vi "Get position.vi"(0 "Zaber":T1={"Serial port handle"="", "Axis"="", "Controller #"=0, "Min position"=0.0, "Max position"=0.0, "Min velocity"=0.0, "Max velocity"=0.0, "Firmware"="", "Device ID"=0, "Variable event"=refnum, "Variable ref"=refnum, "Resolution, usteps/step"=0, "Serial port semaphore"=refnum, "Joystick buttons"={"MinDir"=1, "MaxDir"=2, "MedSpeed"=5, "HighSpeed"=6}} {"Joystick buttons"."HighSpeed" min=1 max=25 step=1; "Joystick buttons"."MedSpeed" min=1 max=25 step=1; "Joystick buttons"."MaxDir" min=1 max=25 step=1; "Joystick buttons"."MinDir" min=1 max=25 step=1}, 5 "error in":errorcluster) -> (11 "Command time, ms":u32, 14 "Zaber out":T1={"Serial port handle"="", "Axis"="", "Controller #"=0, "Min position"=0.0, "Max position"=0.0, "Min velocity"=0.0, "Max velocity"=0.0, "Firmware"="", "Device ID"=0, "Variable event"=refnum, "Variable ref"=refnum, "Resolution, usteps/step"=0, "Serial port semaphore"=refnum, "Joystick buttons"={"MinDir"=1, "MaxDir"=2, "MedSpeed"=5, "HighSpeed"=6}} {"Joystick buttons"."HighSpeed" min=1 max=25 step=1; "Joystick buttons"."MedSpeed" min=1 max=25 step=1; "Joystick buttons"."MaxDir" min=1 max=25 step=1; "Joystick buttons"."MinDir" min=1 max=25 step=1}, 15 "Position, usteps":i32, 16 "PositionRb":dbl caption="Position, mm", 19 "error out":errorcluster)   [LabVIEW 2018]
uses:
  Zaber.ctl
  GenericDataEvent/GenericEvent.ctl
  ZaberVariables.ctl
  CommandZaber.ctl
  GenericDataEvent/GenericData.ctl
panel:
  out "x-y 2":u32
  out "x-y":u32
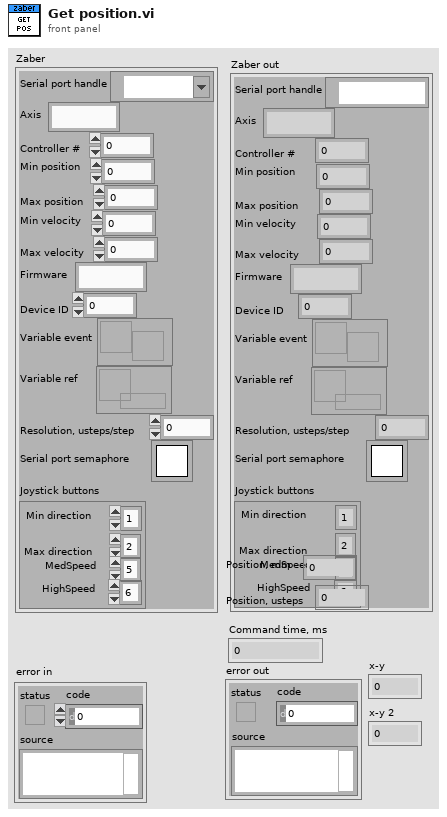
[diagram p1: front panel]
types:
  T1 = typedef "Zaber.ctl" = cluster{"Serial port handle":refnum<visa-resource-name>, "Axis":string, "Controller #":u8, "Min position":dbl, "Max position":dbl, "Min velocity":dbl, "Max velocity":dbl, "Firmware":string, "Device ID":i32, "Variable event":T2, "Variable ref":refnum<data-value>, "Resolution, usteps/step":i32, "Serial port semaphore":T3, "Joystick buttons":cluster{"MinDir":i32, "MaxDir":i32, "MedSpeed":i32, "HighSpeed":i32}}
  T2 = typedef "GenericEvent.ctl" = refnum<user-event>
  T3 = typedef "Semaphore RefNum" = refnum<k1>
  T4 = typedef "CommandZaber.ctl" = cluster{"Command":u8, "Data":i32}
  T5 = typedef "ZaberVariables.ctl" = cluster{"Position":i32, "Speed":i32, "Min soft position":dbl, "Max soft position":dbl, "Accelaration":i32}
  T6 = typedef "GenericData.ctl" = cluster{"Name":string, "Data":variant}
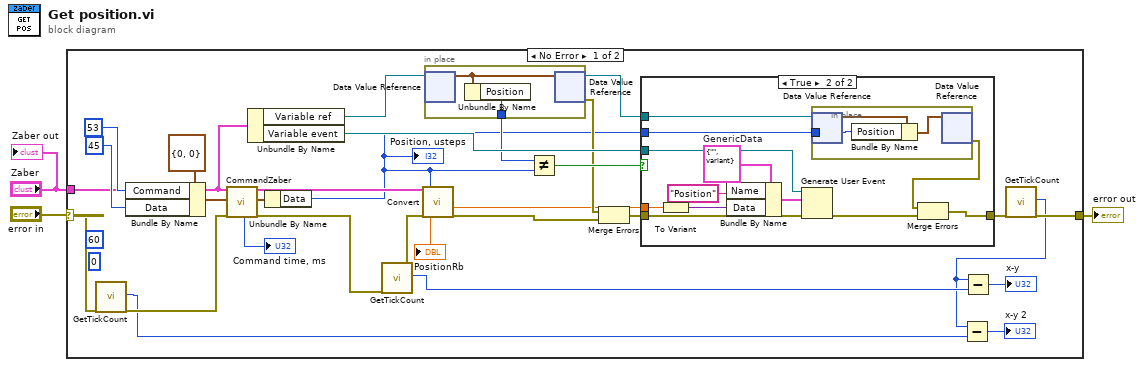
[diagram p0: block diagram]
diagram:
  n1 = case shown="No Error" "error in" {
    selector: "error in" -> [w8 w51]
    tunnel: [w13 w51] -> w2
    tunnel: "Zaber" -> [w24 _]
    frame No Error {
      (unwired) 60 ("Data")
      (unwired) 0 ("Data")
      n2 = call "GetTickCount.vi"("error in (no error)"=w8) -> ("ms"=w5:u32, "error IO"=w7:errorcluster)  [unwired: 17 in]
      n3 = Bundle By Name(cluster=T4 {"Command"=0, "Data"=0} ("Command"), "Command"=53 ("Data"), "Data"=45) -> (w30:T4)
      n4 = call "CommandZaber.vi"("Zaber"=w24, "Command"=w30, "error in"=w7) -> ("Command time, ms"=→"Command time, ms":u32, "Zaber out"=w18:T1, "Answer"=w28:T4, "error out"=w12:errorcluster)  [unwired: 13 in]
      n5 = Unbundle By Name(w24) -> ("Variable ref"=w23:refnum<data-value>, "Variable event"=w26:T2)
      n6 = Unbundle By Name(w28) -> ("Data"=w17:i32)
      "Position, usteps" <- w17
      n7 = call "GetTickCount.vi"("error in (no error)"=w12) -> ("ms"=w10:u32, "error IO"=w11:errorcluster)  [unwired: 17 in]
      n8 = call "Convert.vi"("Zaber"=w18, "error in"=w11, "Position, usteps"=w17) -> ("Position, mm"=w15:dbl, "error out"=w16:errorcluster)  [unwired: 8 in, 7 out]
      "PositionRb" <- w15
      n9 = in-place {
        in-place-border: [w33] -> w21
        n10 = in-place-dvr #1(w23) -> (w34:T5)  [unwired: 1 out]
        n11 = Unbundle By Name(w34) -> ("Position"=w33:i32)
        n12 = in-place-dvr #1(w34) -> (w22:refnum<data-value>, w20:errorcluster)
      }
      n13 = Not Equal?(x=w21, y=w17) -> (x != y?=w25:bool)
      n14 = Merge Errors(w20, w16) -> (w19:errorcluster)
      n15 = case shown="True" w25 {
        tunnel: [w35 w37] -> w14
        tunnel: w15 -> [_ w47]
        tunnel: w19 -> [w35 w45]
        tunnel: w26 -> [_ w46]
        tunnel: w17 -> [_ w39]
        tunnel: w22 -> [_ w40]
        frame False {
        }
        frame True {
          w43 = T6 {"Name"="", "Data"=variant}  # GenericData
          n16 = To Variant(anything=w47) -> (Variant=w42:variant)
          n17 = Bundle By Name(cluster=w43, "Name"="Position" ("Parameter"), "Data"=w42) -> (w41:T6)
          n18 = Generate User Event(user event=w46, event data cluster=w41, error in=w45) -> (error out=w38:errorcluster)  [unwired: 1 in, 1 out]
          n19 = in-place {
            in-place-border: w39 -> [w50]
            n20 = in-place-dvr #2(w40) -> (w49:T5)  [unwired: 1 out]
            n21 = Bundle By Name(cluster=w49, "Position"=w50) -> (w48:T5)
            n22 = in-place-dvr #2(w48) -> (w36:errorcluster)  [unwired: 1 out]
          }
          n23 = Merge Errors(w36, w38) -> (w37:errorcluster)
        }
      }
      n24 = call "GetTickCount.vi"("error in (no error)"=w14) -> ("ms"=w6:u32, "error IO"=w13:errorcluster)  [unwired: 17 in]
      n25 = Subtract(x=w6, y=w5) -> (x-y=→"x-y 2":u32)
      n26 = Subtract(x=w6, y=w10) -> (x-y=→"x-y":u32)
    }
    frame Error {
    }
  }
  "error out" <- w2
  "Zaber out" <- "Zaber"
